vi "Klinger ConvUnit.vi"   [LabVIEW 2010]
doc: "Ce VI convertit le nombre spécifié de l'unitée actuelle vers l'unité demandée. Les différentes unité de déplacement disponible sont les pas, les µm et les picosecondes."
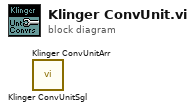
[diagram p0: block diagram]
diagram:
  n1 = call <userlib>:"Klinger ConvUnitSgl.vi"() -> ()  [unwired: 14 in, 2 out]
  n2 = call <userlib>:"Klinger ConvUnitArr.vi"() -> ()  [unwired: 14 in, 2 out]
